vi "dosimat_execute_method.vi"(2 "error in":errorcluster, 3 "Dosimat Port In":refnum<visa-resource-name>="COM1") -> (0 "error out":errorcluster, 1 "Dosimat Port Out":refnum<visa-resource-name>="COM1")   [LabVIEW 2010]
panel:
  # "mooseNote: executes a method that has previously been\nsent to the 876 using the 876 Load Method.vi"
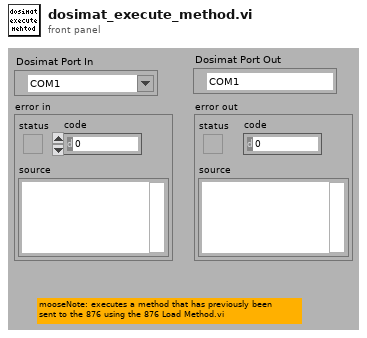
[diagram p1: front panel]
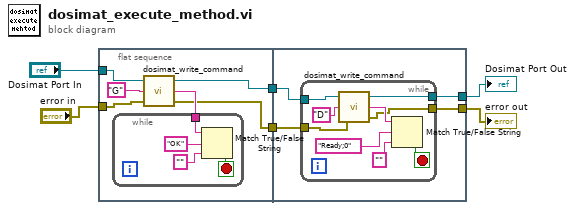
[diagram p0: block diagram]
diagram:
  n1 = flat-sequence {
    tunnel: "Dosimat Port In" -> [w10]
    tunnel: [w9] -> w5
    tunnel: [w8] -> w4
    tunnel: "error in" -> [w7]
    tunnel: w5 -> [w20]
    tunnel: w4 -> [w19]
    tunnel: [w18] -> w2
    tunnel: [w17] -> w1
    frame #0 {
      n2 = call "dosimat_write_command.vi"("error in"=w7, "write buffer"="G", "Dosimat Port In"=w10) -> ("error out"=w8:errorcluster, "read buffer"=w11:string, "Dosimat Port Out"=w9:refnum<visa-resource-name>)
      n3 = while {
        tunnel: w11 -> [w13]
        stop <- w14 stop-if-true
        n4 = Match True/False String(2:"" ("false string"), 3:"OK" ("true string"), 4:w13) -> (0:w14:bool)  [unwired: 1 out]
      }
    }
    frame #1 {
      n5 = while {
        tunnel: w20 -> [w24]
        tunnel: w19 -> [w23]
        tunnel: [w22] -> w18
        tunnel: [w21] -> w17
        stop <- w27 stop-if-true
        n6 = call "dosimat_write_command.vi"("error in"=w23, "write buffer"="D", "Dosimat Port In"=w24) -> ("error out"=w21:errorcluster, "read buffer"=w25:string, "Dosimat Port Out"=w22:refnum<visa-resource-name>)
        n7 = Match True/False String(2:"" ("false string"), 3:"Ready;0" ("true string"), 4:w25) -> (0:w27:bool)  [unwired: 1 out]
      }
    }
  }
  "error out" <- w1
  "Dosimat Port Out" <- w2
